vi "MV3D RGBD Get U3Device List.vi"(10 "nMaxDeviceCount":u32) -> (0 "pDeviceCount out":u32, 1 "MV3D_RGBD_GigEDEVICE_ByteINFO out 2":T1(array[cluster]), 2 "MV3D_RGBD_GigEDEVICE_INFO out 2":T2(array[cluster]), 3 "function return":i32)   [LabVIEW 2015, in "Mv3dRgbdEx.lvlib"]
doc: "MV3D_RGBD_API_Ex MV3D_RGBD_STATUS MV3D_RGBD_GetU3DeviceList(MV3D_RGBD_U3DEVICE_INFO* pstU3DeviceInfos, uint32_t nMaxDeviceCount, uint32_t* pDeviceCount);"
uses:
  <userlib>/Mv3dRgbdEx/Mv3dRgbdEx.lvlib
  <userlib>/Mv3dRgbdEx/Mv3dRgbdEx.dll
panel:
  in  "pstU3DeviceInfos 2":u8[](array[numeric])
  in  "pDeviceCount":u32
types:
  T1 = cluster{"chManufacturerName[0]":i8, "chManufacturerName[1]":i8, "chManufacturerName[2]":i8, "chManufacturerName[3]":i8, "chManufacturerName[4]":i8, "chManufacturerName[5]":i8, "chManufacturerName[6]":i8, "chManufacturerName[7]":i8, "chManufacturerName[8]":i8, "chManufacturerName[9]":i8, "chManufacturerName[10]":i8, "chManufacturerName[11]":i8, "chManufacturerName[12]":i8, "chManufacturerName[13]":i8, "chManufacturerName[14]":i8, "chManufacturerName[15]":i8, "chManufacturerName[16]":i8, "chManufacturerName[17]":i8, "chManufacturerName[18]":i8, "chManufacturerName[19]":i8, "chManufacturerName[20]":i8, "chManufacturerName[21]":i8, "chManufacturerName[22]":i8, "chManufacturerName[23]":i8, "chManufacturerName[24]":i8, "chManufacturerName[25]":i8, "chManufacturerName[26]":i8, "chManufacturerName[27]":i8, "chManufacturerName[28]":i8, "chManufacturerName[29]":i8, "chManufacturerName[30]":i8, "chManufacturerName[31]":i8, "chModelName[0]":i8, "chModelName[1]":i8, "chModelName[2]":i8, "chModelName[3]":i8, "chModelName[4]":i8, "chModelName[5]":i8, "chModelName[6]":i8, "chModelName[7]":i8, "chModelName[8]":i8, "chModelName[9]":i8, "chModelName[10]":i8, "chModelName[11]":i8, "chModelName[12]":i8, "chModelName[13]":i8, "chModelName[14]":i8, "chModelName[15]":i8, "chModelName[16]":i8, "chModelName[17]":i8, "chModelName[18]":i8, "chModelName[19]":i8, "chModelName[20]":i8, "chModelName[21]":i8, "chModelName[22]":i8, "chModelName[23]":i8, "chModelName[24]":i8, "chModelName[25]":i8, "chModelName[26]":i8, "chModelName[27]":i8, "chModelName[28]":i8, "chModelName[29]":i8, "chModelName[30]":i8, "chModelName[31]":i8, "chDeviceVersion[0]":i8, "chDeviceVersion[1]":i8, "chDeviceVersion[2]":i8, "chDeviceVersion[3]":i8, "chDeviceVersion[4]":i8, "chDeviceVersion[5]":i8, "chDeviceVersion[6]":i8, "chDeviceVersion[7]":i8, "chDeviceVersion[8]":i8, "chDeviceVersion[9]":i8, "chDeviceVersion[10]":i8, "chDeviceVersion[11]":i8, "chDeviceVersion[12]":i8, "chDeviceVersion[13]":i8, "chDeviceVersion[14]":i8, "chDeviceVersion[15]":i8, "chDeviceVersion[16]":i8, "chDeviceVersion[17]":i8, "chDeviceVersion[18]":i8, "chDeviceVersion[19]":i8, "chDeviceVersion[20]":i8, "chDeviceVersion[21]":i8, "chDeviceVersion[22]":i8, "chDeviceVersion[23]":i8, "chDeviceVersion[24]":i8, "chDeviceVersion[25]":i8, "chDeviceVersion[26]":i8, "chDeviceVersion[27]":i8, "chDeviceVersion[28]":i8, "chDeviceVersion[29]":i8, "chDeviceVersion[30]":i8, "chDeviceVersion[31]":i8, "chManufacturerSpecificInfo[0]":i8, "chManufacturerSpecificInfo[1]":i8, "chManufacturerSpecificInfo[2]":i8, "chManufacturerSpecificInfo[3]":i8, "chManufacturerSpecificInfo[4]":i8, "chManufacturerSpecificInfo[5]":i8, "chManufacturerSpecificInfo[6]":i8, "chManufacturerSpecificInfo[7]":i8, "chManufacturerSpecificInfo[8]":i8, "chManufacturerSpecificInfo[9]":i8, "chManufacturerSpecificInfo[10]":i8, "chManufacturerSpecificInfo[11]":i8, "chManufacturerSpecificInfo[12]":i8, "chManufacturerSpecificInfo[13]":i8, "chManufacturerSpecificInfo[14]":i8, "chManufacturerSpecificInfo[15]":i8, "chManufacturerSpecificInfo[16]":i8, "chManufacturerSpecificInfo[17]":i8, "chManufacturerSpecificInfo[18]":i8, "chManufacturerSpecificInfo[19]":i8, "chManufacturerSpecificInfo[20]":i8, "chManufacturerSpecificInfo[21]":i8, "chManufacturerSpecificInfo[22]":i8, "chManufacturerSpecificInfo[23]":i8, "chManufacturerSpecificInfo[24]":i8, "chManufacturerSpecificInfo[25]":i8, "chManufacturerSpecificInfo[26]":i8, "chManufacturerSpecificInfo[27]":i8, "chManufacturerSpecificInfo[28]":i8, "chManufacturerSpecificInfo[29]":i8, "chManufacturerSpecificInfo[30]":i8, "chManufacturerSpecificInfo[31]":i8, "chManufacturerSpecificInfo[32]":i8, "chManufacturerSpecificInfo[33]":i8, "chManufacturerSpecificInfo[34]":i8, "chManufacturerSpecificInfo[35]":i8, "chManufacturerSpecificInfo[36]":i8, "chManufacturerSpecificInfo[37]":i8, "chManufacturerSpecificInfo[38]":i8, "chManufacturerSpecificInfo[39]":i8, "chManufacturerSpecificInfo[40]":i8, "chManufacturerSpecificInfo[41]":i8, "chManufacturerSpecificInfo[42]":i8, "chManufacturerSpecificInfo[43]":i8, "chManufacturerSpecificInfo[44]":i8, "chManufacturerSpecificInfo[45]":i8, "chManufacturerSpecificInfo[46]":i8, "chManufacturerSpecificInfo[47]":i8, "chSerialNumber[0]":i8, "chSerialNumber[1]":i8, "chSerialNumber[2]":i8, "chSerialNumber[3]":i8, "chSerialNumber[4]":i8, "chSerialNumber[5]":i8, "chSerialNumber[6]":i8, "chSerialNumber[7]":i8, "chSerialNumber[8]":i8, "chSerialNumber[9]":i8, "chSerialNumber[10]":i8, "chSerialNumber[11]":i8, "chSerialNumber[12]":i8, "chSerialNumber[13]":i8, "chSerialNumber[14]":i8, "chSerialNumber[15]":i8, "chUserDefinedName[0]":i8, "chUserDefinedName[1]":i8, "chUserDefinedName[2]":i8, "chUserDefinedName[3]":i8, "chUserDefinedName[4]":i8, "chUserDefinedName[5]":i8, "chUserDefinedName[6]":i8, "chUserDefinedName[7]":i8, "chUserDefinedName[8]":i8, "chUserDefinedName[9]":i8, "chUserDefinedName[10]":i8, "chUserDefinedName[11]":i8, "chUserDefinedName[12]":i8, "chUserDefinedName[13]":i8, "chUserDefinedName[14]":i8, "chUserDefinedName[15]":i8, "enDeviceType":i32, "nVendorId":u32, "nProductId":u32, "enUsbProtocol":i32, "chDeviceGUID[0]":i8, "chDeviceGUID[1]":i8, "chDeviceGUID[2]":i8, "chDeviceGUID[3]":i8, "chDeviceGUID[4]":i8, "chDeviceGUID[5]":i8, "chDeviceGUID[6]":i8, "chDeviceGUID[7]":i8, "chDeviceGUID[8]":i8, "chDeviceGUID[9]":i8, "chDeviceGUID[10]":i8, "chDeviceGUID[11]":i8, "chDeviceGUID[12]":i8, "chDeviceGUID[13]":i8, "chDeviceGUID[14]":i8, "chDeviceGUID[15]":i8, "chDeviceGUID[16]":i8, "chDeviceGUID[17]":i8, "chDeviceGUID[18]":i8, "chDeviceGUID[19]":i8, "chDeviceGUID[20]":i8, "chDeviceGUID[21]":i8, "chDeviceGUID[22]":i8, "chDeviceGUID[23]":i8, "chDeviceGUID[24]":i8, "chDeviceGUID[25]":i8, "chDeviceGUID[26]":i8, "chDeviceGUID[27]":i8, "chDeviceGUID[28]":i8, "chDeviceGUID[29]":i8, "chDeviceGUID[30]":i8, "chDeviceGUID[31]":i8, "chDeviceGUID[32]":i8, "chDeviceGUID[33]":i8, "chDeviceGUID[34]":i8, "chDeviceGUID[35]":i8, "chDeviceGUID[36]":i8, "chDeviceGUID[37]":i8, "chDeviceGUID[38]":i8, "chDeviceGUID[39]":i8, "chDeviceGUID[40]":i8, "chDeviceGUID[41]":i8, "chDeviceGUID[42]":i8, "chDeviceGUID[43]":i8, "chDeviceGUID[44]":i8, "chDeviceGUID[45]":i8, "chDeviceGUID[46]":i8, "chDeviceGUID[47]":i8, "chDeviceGUID[48]":i8, "chDeviceGUID[49]":i8, "chDeviceGUID[50]":i8, "chDeviceGUID[51]":i8, "chDeviceGUID[52]":i8, "chDeviceGUID[53]":i8, "chDeviceGUID[54]":i8, "chDeviceGUID[55]":i8, "chDeviceGUID[56]":i8, "chDeviceGUID[57]":i8, "chDeviceGUID[58]":i8, "chDeviceGUID[59]":i8, "chDeviceGUID[60]":i8, "chDeviceGUID[61]":i8, "chDeviceGUID[62]":i8, "chDeviceGUID[63]":i8, "nReserved[0]":u8, "nReserved[1]":u8, "nReserved[2]":u8, "nReserved[3]":u8, "nReserved[4]":u8, "nReserved[5]":u8, "nReserved[6]":u8, "nReserved[7]":u8, "nReserved[8]":u8, "nReserved[9]":u8, "nReserved[10]":u8, "nReserved[11]":u8, "nReserved[12]":u8, "nReserved[13]":u8, "nReserved[14]":u8, "nReserved[15]":u8}[]
  T2 = cluster{"chManufacturerName":string, "chModelName":string, "chDeviceVersion":string, "chManufacturerSpecificInfo":string, "chSerialNumber":u8[], "chUserDefinedName":string, "enDeviceType":i32, "nVendorId":u32, "nProductId":u32, "enUsbProtocol":i32, "chDeviceGUID":string, "nReserved":string}[]
  T3 = cluster{"chManufacturerName[0]":i8, "chManufacturerName[1]":i8, "chManufacturerName[2]":i8, "chManufacturerName[3]":i8, "chManufacturerName[4]":i8, "chManufacturerName[5]":i8, "chManufacturerName[6]":i8, "chManufacturerName[7]":i8, "chManufacturerName[8]":i8, "chManufacturerName[9]":i8, "chManufacturerName[10]":i8, "chManufacturerName[11]":i8, "chManufacturerName[12]":i8, "chManufacturerName[13]":i8, "chManufacturerName[14]":i8, "chManufacturerName[15]":i8, "chManufacturerName[16]":i8, "chManufacturerName[17]":i8, "chManufacturerName[18]":i8, "chManufacturerName[19]":i8, "chManufacturerName[20]":i8, "chManufacturerName[21]":i8, "chManufacturerName[22]":i8, "chManufacturerName[23]":i8, "chManufacturerName[24]":i8, "chManufacturerName[25]":i8, "chManufacturerName[26]":i8, "chManufacturerName[27]":i8, "chManufacturerName[28]":i8, "chManufacturerName[29]":i8, "chManufacturerName[30]":i8, "chManufacturerName[31]":i8, "chModelName[0]":i8, "chModelName[1]":i8, "chModelName[2]":i8, "chModelName[3]":i8, "chModelName[4]":i8, "chModelName[5]":i8, "chModelName[6]":i8, "chModelName[7]":i8, "chModelName[8]":i8, "chModelName[9]":i8, "chModelName[10]":i8, "chModelName[11]":i8, "chModelName[12]":i8, "chModelName[13]":i8, "chModelName[14]":i8, "chModelName[15]":i8, "chModelName[16]":i8, "chModelName[17]":i8, "chModelName[18]":i8, "chModelName[19]":i8, "chModelName[20]":i8, "chModelName[21]":i8, "chModelName[22]":i8, "chModelName[23]":i8, "chModelName[24]":i8, "chModelName[25]":i8, "chModelName[26]":i8, "chModelName[27]":i8, "chModelName[28]":i8, "chModelName[29]":i8, "chModelName[30]":i8, "chModelName[31]":i8, "chDeviceVersion[0]":i8, "chDeviceVersion[1]":i8, "chDeviceVersion[2]":i8, "chDeviceVersion[3]":i8, "chDeviceVersion[4]":i8, "chDeviceVersion[5]":i8, "chDeviceVersion[6]":i8, "chDeviceVersion[7]":i8, "chDeviceVersion[8]":i8, "chDeviceVersion[9]":i8, "chDeviceVersion[10]":i8, "chDeviceVersion[11]":i8, "chDeviceVersion[12]":i8, "chDeviceVersion[13]":i8, "chDeviceVersion[14]":i8, "chDeviceVersion[15]":i8, "chDeviceVersion[16]":i8, "chDeviceVersion[17]":i8, "chDeviceVersion[18]":i8, "chDeviceVersion[19]":i8, "chDeviceVersion[20]":i8, "chDeviceVersion[21]":i8, "chDeviceVersion[22]":i8, "chDeviceVersion[23]":i8, "chDeviceVersion[24]":i8, "chDeviceVersion[25]":i8, "chDeviceVersion[26]":i8, "chDeviceVersion[27]":i8, "chDeviceVersion[28]":i8, "chDeviceVersion[29]":i8, "chDeviceVersion[30]":i8, "chDeviceVersion[31]":i8, "chManufacturerSpecificInfo[0]":i8, "chManufacturerSpecificInfo[1]":i8, "chManufacturerSpecificInfo[2]":i8, "chManufacturerSpecificInfo[3]":i8, "chManufacturerSpecificInfo[4]":i8, "chManufacturerSpecificInfo[5]":i8, "chManufacturerSpecificInfo[6]":i8, "chManufacturerSpecificInfo[7]":i8, "chManufacturerSpecificInfo[8]":i8, "chManufacturerSpecificInfo[9]":i8, "chManufacturerSpecificInfo[10]":i8, "chManufacturerSpecificInfo[11]":i8, "chManufacturerSpecificInfo[12]":i8, "chManufacturerSpecificInfo[13]":i8, "chManufacturerSpecificInfo[14]":i8, "chManufacturerSpecificInfo[15]":i8, "chManufacturerSpecificInfo[16]":i8, "chManufacturerSpecificInfo[17]":i8, "chManufacturerSpecificInfo[18]":i8, "chManufacturerSpecificInfo[19]":i8, "chManufacturerSpecificInfo[20]":i8, "chManufacturerSpecificInfo[21]":i8, "chManufacturerSpecificInfo[22]":i8, "chManufacturerSpecificInfo[23]":i8, "chManufacturerSpecificInfo[24]":i8, "chManufacturerSpecificInfo[25]":i8, "chManufacturerSpecificInfo[26]":i8, "chManufacturerSpecificInfo[27]":i8, "chManufacturerSpecificInfo[28]":i8, "chManufacturerSpecificInfo[29]":i8, "chManufacturerSpecificInfo[30]":i8, "chManufacturerSpecificInfo[31]":i8, "chManufacturerSpecificInfo[32]":i8, "chManufacturerSpecificInfo[33]":i8, "chManufacturerSpecificInfo[34]":i8, "chManufacturerSpecificInfo[35]":i8, "chManufacturerSpecificInfo[36]":i8, "chManufacturerSpecificInfo[37]":i8, "chManufacturerSpecificInfo[38]":i8, "chManufacturerSpecificInfo[39]":i8, "chManufacturerSpecificInfo[40]":i8, "chManufacturerSpecificInfo[41]":i8, "chManufacturerSpecificInfo[42]":i8, "chManufacturerSpecificInfo[43]":i8, "chManufacturerSpecificInfo[44]":i8, "chManufacturerSpecificInfo[45]":i8, "chManufacturerSpecificInfo[46]":i8, "chManufacturerSpecificInfo[47]":i8, "chSerialNumber[0]":i8, "chSerialNumber[1]":i8, "chSerialNumber[2]":i8, "chSerialNumber[3]":i8, "chSerialNumber[4]":i8, "chSerialNumber[5]":i8, "chSerialNumber[6]":i8, "chSerialNumber[7]":i8, "chSerialNumber[8]":i8, "chSerialNumber[9]":i8, "chSerialNumber[10]":i8, "chSerialNumber[11]":i8, "chSerialNumber[12]":i8, "chSerialNumber[13]":i8, "chSerialNumber[14]":i8, "chSerialNumber[15]":i8, "chUserDefinedName[0]":i8, "chUserDefinedName[1]":i8, "chUserDefinedName[2]":i8, "chUserDefinedName[3]":i8, "chUserDefinedName[4]":i8, "chUserDefinedName[5]":i8, "chUserDefinedName[6]":i8, "chUserDefinedName[7]":i8, "chUserDefinedName[8]":i8, "chUserDefinedName[9]":i8, "chUserDefinedName[10]":i8, "chUserDefinedName[11]":i8, "chUserDefinedName[12]":i8, "chUserDefinedName[13]":i8, "chUserDefinedName[14]":i8, "chUserDefinedName[15]":i8, "enDeviceType":i32, "nVendorId":u32, "nProductId":u32, "enUsbProtocol":i32, "chDeviceGUID[0]":i8, "chDeviceGUID[1]":i8, "chDeviceGUID[2]":i8, "chDeviceGUID[3]":i8, "chDeviceGUID[4]":i8, "chDeviceGUID[5]":i8, "chDeviceGUID[6]":i8, "chDeviceGUID[7]":i8, "chDeviceGUID[8]":i8, "chDeviceGUID[9]":i8, "chDeviceGUID[10]":i8, "chDeviceGUID[11]":i8, "chDeviceGUID[12]":i8, "chDeviceGUID[13]":i8, "chDeviceGUID[14]":i8, "chDeviceGUID[15]":i8, "chDeviceGUID[16]":i8, "chDeviceGUID[17]":i8, "chDeviceGUID[18]":i8, "chDeviceGUID[19]":i8, "chDeviceGUID[20]":i8, "chDeviceGUID[21]":i8, "chDeviceGUID[22]":i8, "chDeviceGUID[23]":i8, "chDeviceGUID[24]":i8, "chDeviceGUID[25]":i8, "chDeviceGUID[26]":i8, "chDeviceGUID[27]":i8, "chDeviceGUID[28]":i8, "chDeviceGUID[29]":i8, "chDeviceGUID[30]":i8, "chDeviceGUID[31]":i8, "chDeviceGUID[32]":i8, "chDeviceGUID[33]":i8, "chDeviceGUID[34]":i8, "chDeviceGUID[35]":i8, "chDeviceGUID[36]":i8, "chDeviceGUID[37]":i8, "chDeviceGUID[38]":i8, "chDeviceGUID[39]":i8, "chDeviceGUID[40]":i8, "chDeviceGUID[41]":i8, "chDeviceGUID[42]":i8, "chDeviceGUID[43]":i8, "chDeviceGUID[44]":i8, "chDeviceGUID[45]":i8, "chDeviceGUID[46]":i8, "chDeviceGUID[47]":i8, "chDeviceGUID[48]":i8, "chDeviceGUID[49]":i8, "chDeviceGUID[50]":i8, "chDeviceGUID[51]":i8, "chDeviceGUID[52]":i8, "chDeviceGUID[53]":i8, "chDeviceGUID[54]":i8, "chDeviceGUID[55]":i8, "chDeviceGUID[56]":i8, "chDeviceGUID[57]":i8, "chDeviceGUID[58]":i8, "chDeviceGUID[59]":i8, "chDeviceGUID[60]":i8, "chDeviceGUID[61]":i8, "chDeviceGUID[62]":i8, "chDeviceGUID[63]":i8, "nReserved[0]":u8, "nReserved[1]":u8, "nReserved[2]":u8, "nReserved[3]":u8, "nReserved[4]":u8, "nReserved[5]":u8, "nReserved[6]":u8, "nReserved[7]":u8, "nReserved[8]":u8, "nReserved[9]":u8, "nReserved[10]":u8, "nReserved[11]":u8, "nReserved[12]":u8, "nReserved[13]":u8, "nReserved[14]":u8, "nReserved[15]":u8}
  T4 = cluster{"chManufacturerName":string, "chModelName":string, "chDeviceVersion":string, "chManufacturerSpecificInfo":string, "chSerialNumber":u8[], "chUserDefinedName":string, "enDeviceType":i32, "nVendorId":u32, "nProductId":u32, "enUsbProtocol":i32, "chDeviceGUID":string, "nReserved":string}
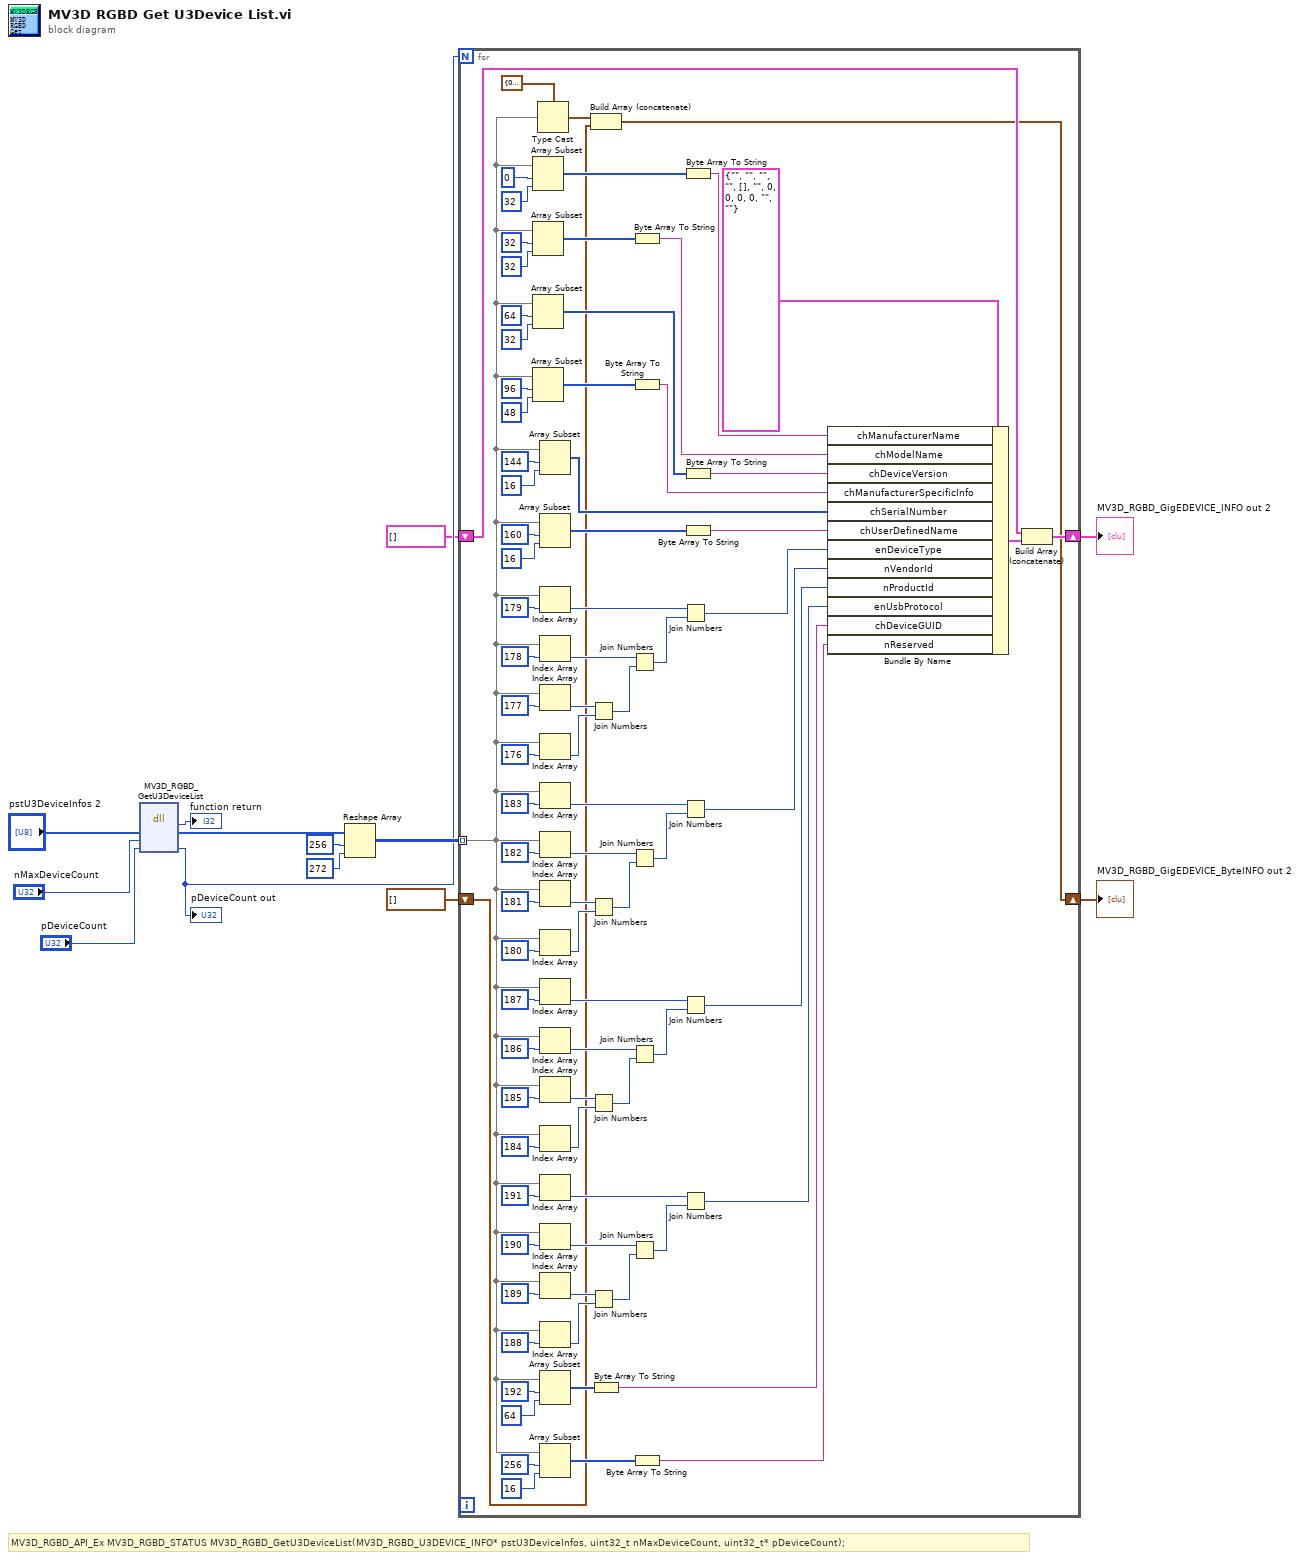
[diagram p0: block diagram]
diagram:
  # "MV3D_RGBD_API_Ex MV3D_RGBD_STATUS MV3D_RGBD_GetU3DeviceList(MV3D_RGBD_U3DEVICE_INFO* pstU3DeviceInfos, uint32_t nMaxDeviceCount, uint32_t* pDeviceCount);"
  n1 = dll-call lib="C:/Program Files (x86)/National Instruments/LabVIEW 2015/user.lib/Mv3dRgbdEx/Mv3dRgbdEx.*" fn="MV3D_RGBD_GetU3DeviceList"("pstU3DeviceInfos"="pstU3DeviceInfos 2", "nMaxDeviceCount"="nMaxDeviceCount", "pDeviceCount"="pDeviceCount") -> ("返回类型"=→"function return":i32, "pstU3DeviceInfos"=w6:u8[], "pDeviceCount"=w5:u32)  [unwired: 4 in, 2 out]
  "pDeviceCount out" <- w5
  n2 = Reshape Array(w6, 256 ("维数大小"), 272 ("维数大小")) -> (w7:u8[][])
  n3 = for {
    N: w5 -> [_]
    shift-right: [w20] -> w3
    shift-left: T2 [] ("MV3D_RGBD_GigEDEVICE_INFO out") -> [w69]
    tunnel: w7 -> [w17] mode=indexing
    shift-right: [w15] -> w1
    shift-left: T1 [] ("*(类型 *) &x") -> [w14]
    n4 = Array Subset(array=w17, index=0 ("索引"), length=32 ("长度")) -> (w95:u8[])
    n5 = Array Subset(array=w17, index=32 ("索引"), length=32 ("长度")) -> (w92:u8[])
    n6 = Array Subset(array=w17, index=64 ("索引"), length=32 ("长度")) -> (w85:u8[])
    n7 = Array Subset(array=w17, index=96 ("索引"), length=48 ("长度")) -> (w89:u8[])
    n8 = Type Cast(type=T3 {"chManufacturerName[0]"=0, "chManufacturerName[1]"=0, "chManufacturerName[2]"=0, "chManufacturerName[3]"=0, "chManufacturerName[4]"=0, "chManufacturerName[5]"=0, "chManufacturerName[6]"=0, "chManufacturerName[7]"=0, "chManufacturerName[8]"=0, "chManufacturerName[9]"=0, "chManufacturerName[10]"=0, "chManufacturerName[11]"=0, "chManufacturerName[12]"=0, "chManufacturerName[13]"=0, "chManufacturerName[14]"=0, "chManufacturerName[15]"=0, "chManufacturerName[16]"=0, "chManufacturerName[17]"=0, "chManufacturerName[18]"=0, "chManufacturerName[19]"=0, "chManufacturerName[20]"=0, "chManufacturerName[21]"=0, "chManufacturerName[22]"=0, "chManufacturerName[23]"=0, "chManufacturerName[24]"=0, "chManufacturerName[25]"=0, "chManufacturerName[26]"=0, "chManufacturerName[27]"=0, "chManufacturerName[28]"=0, "chManufacturerName[29]"=0, "chManufacturerName[30]"=0, "chManufacturerName[31]"=0, "chModelName[0]"=0, "chModelName[1]"=0, "chModelName[2]"=0, "chModelName[3]"=0, "chModelName[4]"=0, "chModelName[5]"=0, "chModelName[6]"=0, "chModelName[7]"=0, "chModelName[8]"=0, "chModelName[9]"=0, "chModelName[10]"=0, "chModelName[11]"=0, "chModelName[12]"=0, "chModelName[13]"=0, "chModelName[14]"=0, "chModelName[15]"=0, "chModelName[16]"=0, "chModelName[17]"=0, "chModelName[18]"=0, "chModelName[19]"=0, "chModelName[20]"=0, "chModelName[21]"=0, "chModelName[22]"=0, "chModelName[23]"=0, "chModelName[24]"=0, "chModelName[25]"=0, "chModelName[26]"=0, "chModelName[27]"=0, "chModelName[28]"=0, "chModelName[29]"=0, "chModelName[30]"=0, "chModelName[31]"=0, "chDeviceVersion[0]"=0, "chDeviceVersion[1]"=0, "chDeviceVersion[2]"=0, "chDeviceVersion[3]"=0, "chDeviceVersion[4]"=0, "chDeviceVersion[5]"=0, "chDeviceVersion[6]"=0, "chDeviceVersion[7]"=0, "chDeviceVersion[8]"=0, "chDeviceVersion[9]"=0, "chDeviceVersion[10]"=0, "chDeviceVersion[11]"=0, "chDeviceVersion[12]"=0, "chDeviceVersion[13]"=0, "chDeviceVersion[14]"=0, "chDeviceVersion[15]"=0, "chDeviceVersion[16]"=0, "chDeviceVersion[17]"=0, "chDeviceVersion[18]"=0, "chDeviceVersion[19]"=0, "chDeviceVersion[20]"=0, "chDeviceVersion[21]"=0, "chDeviceVersion[22]"=0, "chDeviceVersion[23]"=0, "chDeviceVersion[24]"=0, "chDeviceVersion[25]"=0, "chDeviceVersion[26]"=0, "chDeviceVersion[27]"=0, "chDeviceVersion[28]"=0, "chDeviceVersion[29]"=0, "chDeviceVersion[30]"=0, "chDeviceVersion[31]"=0, "chManufacturerSpecificInfo[0]"=0, "chManufacturerSpecificInfo[1]"=0, "chManufacturerSpecificInfo[2]"=0, "chManufacturerSpecificInfo[3]"=0, "chManufacturerSpecificInfo[4]"=0, "chManufacturerSpecificInfo[5]"=0, "chManufacturerSpecificInfo[6]"=0, "chManufacturerSpecificInfo[7]"=0, "chManufacturerSpecificInfo[8]"=0, "chManufacturerSpecificInfo[9]"=0, "chManufacturerSpecificInfo[10]"=0, "chManufacturerSpecificInfo[11]"=0, "chManufacturerSpecificInfo[12]"=0, "chManufacturerSpecificInfo[13]"=0, "chManufacturerSpecificInfo[14]"=0, "chManufacturerSpecificInfo[15]"=0, "chManufacturerSpecificInfo[16]"=0, "chManufacturerSpecificInfo[17]"=0, "chManufacturerSpecificInfo[18]"=0, "chManufacturerSpecificInfo[19]"=0, "chManufacturerSpecificInfo[20]"=0, "chManufacturerSpecificInfo[21]"=0, "chManufacturerSpecificInfo[22]"=0, "chManufacturerSpecificInfo[23]"=0, "chManufacturerSpecificInfo[24]"=0, "chManufacturerSpecificInfo[25]"=0, "chManufacturerSpecificInfo[26]"=0, "chManufacturerSpecificInfo[27]"=0, "chManufacturerSpecificInfo[28]"=0, "chManufacturerSpecificInfo[29]"=0, "chManufacturerSpecificInfo[30]"=0, "chManufacturerSpecificInfo[31]"=0, "chManufacturerSpecificInfo[32]"=0, "chManufacturerSpecificInfo[33]"=0, "chManufacturerSpecificInfo[34]"=0, "chManufacturerSpecificInfo[35]"=0, "chManufacturerSpecificInfo[36]"=0, "chManufacturerSpecificInfo[37]"=0, "chManufacturerSpecificInfo[38]"=0, "chManufacturerSpecificInfo[39]"=0, "chManufacturerSpecificInfo[40]"=0, "chManufacturerSpecificInfo[41]"=0, "chManufacturerSpecificInfo[42]"=0, "chManufacturerSpecificInfo[43]"=0, "chManufacturerSpecificInfo[44]"=0, "chManufacturerSpecificInfo[45]"=0, "chManufacturerSpecificInfo[46]"=0, "chManufacturerSpecificInfo[47]"=0, "chSerialNumber[0]"=0, "chSerialNumber[1]"=0, "chSerialNumber[2]"=0, "chSerialNumber[3]"=0, "chSerialNumber[4]"=0, "chSerialNumber[5]"=0, "chSerialNumber[6]"=0, "chSerialNumber[7]"=0, "chSerialNumber[8]"=0, "chSerialNumber[9]"=0, "chSerialNumber[10]"=0, "chSerialNumber[11]"=0, "chSerialNumber[12]"=0, "chSerialNumber[13]"=0, "chSerialNumber[14]"=0, "chSerialNumber[15]"=0, "chUserDefinedName[0]"=0, "chUserDefinedName[1]"=0, "chUserDefinedName[2]"=0, "chUserDefinedName[3]"=0, "chUserDefinedName[4]"=0, "chUserDefinedName[5]"=0, "chUserDefinedName[6]"=0, "chUserDefinedName[7]"=0, "chUserDefinedName[8]"=0, "chUserDefinedName[9]"=0, "chUserDefinedName[10]"=0, "chUserDefinedName[11]"=0, "chUserDefinedName[12]"=0, "chUserDefinedName[13]"=0, "chUserDefinedName[14]"=0, "chUserDefinedName[15]"=0, "enDeviceType"=0, "nVendorId"=0, "nProductId"=0, "enUsbProtocol"=0, "chDeviceGUID[0]"=0, "chDeviceGUID[1]"=0, "chDeviceGUID[2]"=0, "chDeviceGUID[3]"=0, "chDeviceGUID[4]"=0, "chDeviceGUID[5]"=0, "chDeviceGUID[6]"=0, "chDeviceGUID[7]"=0, "chDeviceGUID[8]"=0, "chDeviceGUID[9]"=0, "chDeviceGUID[10]"=0, "chDeviceGUID[11]"=0, "chDeviceGUID[12]"=0, "chDeviceGUID[13]"=0, "chDeviceGUID[14]"=0, "chDeviceGUID[15]"=0, "chDeviceGUID[16]"=0, "chDeviceGUID[17]"=0, "chDeviceGUID[18]"=0, "chDeviceGUID[19]"=0, "chDeviceGUID[20]"=0, "chDeviceGUID[21]"=0, "chDeviceGUID[22]"=0, "chDeviceGUID[23]"=0, "chDeviceGUID[24]"=0, "chDeviceGUID[25]"=0, "chDeviceGUID[26]"=0, "chDeviceGUID[27]"=0, "chDeviceGUID[28]"=0, "chDeviceGUID[29]"=0, "chDeviceGUID[30]"=0, "chDeviceGUID[31]"=0, "chDeviceGUID[32]"=0, "chDeviceGUID[33]"=0, "chDeviceGUID[34]"=0, "chDeviceGUID[35]"=0, "chDeviceGUID[36]"=0, "chDeviceGUID[37]"=0, "chDeviceGUID[38]"=0, "chDeviceGUID[39]"=0, "chDeviceGUID[40]"=0, "chDeviceGUID[41]"=0, "chDeviceGUID[42]"=0, "chDeviceGUID[43]"=0, "chDeviceGUID[44]"=0, "chDeviceGUID[45]"=0, "chDeviceGUID[46]"=0, "chDeviceGUID[47]"=0, "chDeviceGUID[48]"=0, "chDeviceGUID[49]"=0, "chDeviceGUID[50]"=0, "chDeviceGUID[51]"=0, "chDeviceGUID[52]"=0, "chDeviceGUID[53]"=0, "chDeviceGUID[54]"=0, "chDeviceGUID[55]"=0, "chDeviceGUID[56]"=0, "chDeviceGUID[57]"=0, "chDeviceGUID[58]"=0, "chDeviceGUID[59]"=0, "chDeviceGUID[60]"=0, "chDeviceGUID[61]"=0, "chDeviceGUID[62]"=0, "chDeviceGUID[63]"=0, "nReserved[0]"=0, "nReserved[1]"=0, "nReserved[2]"=0, "nReserved[3]"=0, "nReserved[4]"=0, "nReserved[5]"=0, "nReserved[6]"=0, "nReserved[7]"=0, "nReserved[8]"=0, "nReserved[9]"=0, "nReserved[10]"=0, "nReserved[11]"=0, "nReserved[12]"=0, "nReserved[13]"=0, "nReserved[14]"=0, "nReserved[15]"=0} ("pstU3DeviceInfos out"), x=w17) -> (*(type *) &x=w16:T3)
    n9 = Array Subset(array=w17, index=144 ("索引"), length=16 ("长度")) -> (w52:u8[])
    n10 = Array Subset(array=w17, index=160 ("索引"), length=16 ("长度")) -> (w86:u8[])
    n11 = Index Array(array=w17, index=179 ("索引")) -> (element=w47:u8)
    n12 = Index Array(array=w17, index=178 ("索引")) -> (element=w48:u8)
    n13 = Index Array(array=w17, index=177 ("索引")) -> (element=w50:u8)
    n14 = Index Array(array=w17, index=176 ("索引")) -> (element=w51:u8)
    n15 = Index Array(array=w17, index=183 ("索引")) -> (element=w36:u8)
    n16 = Index Array(array=w17, index=182 ("索引")) -> (element=w37:u8)
    n17 = Index Array(array=w17, index=181 ("索引")) -> (element=w39:u8)
    n18 = Index Array(array=w17, index=180 ("索引")) -> (element=w40:u8)
    n19 = Index Array(array=w17, index=187 ("索引")) -> (element=w62:u8)
    n20 = Index Array(array=w17, index=186 ("索引")) -> (element=w60:u8)
    n21 = Index Array(array=w17, index=185 ("索引")) -> (element=w58:u8)
    n22 = Index Array(array=w17, index=184 ("索引")) -> (element=w53:u8)
    n23 = Index Array(array=w17, index=191 ("索引")) -> (element=w25:u8)
    n24 = Index Array(array=w17, index=190 ("索引")) -> (element=w26:u8)
    n25 = Index Array(array=w17, index=189 ("索引")) -> (element=w28:u8)
    n26 = Index Array(array=w17, index=188 ("索引")) -> (element=w29:u8)
    n27 = Array Subset(array=w17, index=192 ("索引"), length=64 ("长度")) -> (w81:u8[])
    n28 = Array Subset(array=w17, index=256 ("索引"), length=16 ("长度")) -> (w79:u8[])
    n29 = Join Numbers(hi=w50, lo=w51) -> ((hi.lo)=w49:u16)
    n30 = Join Numbers(hi=w39, lo=w40) -> ((hi.lo)=w38:u16)
    n31 = Join Numbers(hi=w58, lo=w53) -> ((hi.lo)=w57:u16)
    n32 = Join Numbers(hi=w28, lo=w29) -> ((hi.lo)=w27:u16)
    n33 = Build Array (concatenate)(w16, w14) -> (w15:T1)
    n34 = Byte Array To String(unsigned byte array=w81) -> (string=w22:string)
    n35 = Join Numbers(hi=w48, lo=w49) -> ((hi.lo)=w46:u32)
    n36 = Join Numbers(hi=w37, lo=w38) -> ((hi.lo)=w35:u32)
    n37 = Join Numbers(hi=w60, lo=w57) -> ((hi.lo)=w56:u32)
    n38 = Join Numbers(hi=w26, lo=w27) -> ((hi.lo)=w24:u32)
    n39 = Byte Array To String(unsigned byte array=w92) -> (string=w73:string)
    n40 = Byte Array To String(unsigned byte array=w89) -> (string=w71:string)
    n41 = Byte Array To String(unsigned byte array=w79) -> (string=w21:string)
    n42 = Join Numbers(hi=w47, lo=w46) -> ((hi.lo)=w64:u64)
    n43 = Join Numbers(hi=w36, lo=w35) -> ((hi.lo)=w34:u64)
    n44 = Join Numbers(hi=w62, lo=w56) -> ((hi.lo)=w55:u64)
    n45 = Join Numbers(hi=w25, lo=w24) -> ((hi.lo)=w23:u64)
    n46 = Byte Array To String(unsigned byte array=w95) -> (string=w74:string)
    n47 = Byte Array To String(unsigned byte array=w85) -> (string=w72:string)
    n48 = Byte Array To String(unsigned byte array=w86) -> (string=w70:string)
    n49 = Bundle By Name(cluster=T4 {"chManufacturerName"="", "chModelName"="", "chDeviceVersion"="", "chManufacturerSpecificInfo"="", "chSerialNumber"=[], "chUserDefinedName"="", "enDeviceType"=0, "nVendorId"=0, "nProductId"=0, "enUsbProtocol"=0, "chDeviceGUID"="", "nReserved"=""} ("MV3D_RGBD_GigEDEVICE_INFO out"), "chManufacturerName"=w74, "chModelName"=w73, "chDeviceVersion"=w72, "chManufacturerSpecificInfo"=w71, "chSerialNumber"=w52, "chUserDefinedName"=w70, "enDeviceType"=w64, "nVendorId"=w34, "nProductId"=w55, "enUsbProtocol"=w23, "chDeviceGUID"=w22, "nReserved"=w21) -> (w19:T4)
    n50 = Build Array (concatenate)(w69, w19) -> (w20:T2)
  }
  "MV3D_RGBD_GigEDEVICE_INFO out 2" <- w3
  "MV3D_RGBD_GigEDEVICE_ByteINFO out 2" <- w1
